vi "pump rpm poly.vi"   [LabVIEW 2012]
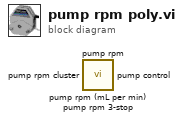
[diagram p0: block diagram]
diagram:
  n1 = call "pump rpm (mL per min).vi"() -> ()  [unwired: 2 in, 4 out]
  n2 = call "pump rpm.vi"() -> ()  [unwired: 2 in, 4 out]
  n3 = call "pump rpm cluster.vi"() -> ()  [unwired: 2 in, 4 out]
  n4 = call <userlib>:"pump control.vi"() -> ()  [unwired: 4 in, 2 out]
  n5 = call "pump rpm 3-stop.vi"() -> ()  [unwired: 4 in, 2 out]
